vi "OpenVIFrontPanel.vi"(0 "VI Reference In":refnum<vi>, 5 "Wait Until Done (F)":bool, 7 "State(Standard)":T1(ring)=enum."Standard", 11 "error in":errorcluster) -> (4 "VI Reference Out":refnum<vi>, 15 "error out":errorcluster)   [LabVIEW 2016, in "Drona.lvlib" / "VI.lvlib"]
doc: "Opens the front panel of the VI by providing the VI reference."
uses:
  VI.lvlib
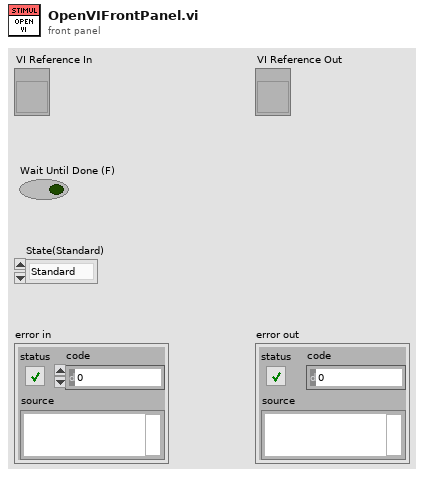
[diagram p1: front panel]
types:
  T1 = enum32{"Invalid", "Standard", "Closed", "Hidden", "Minimized", "Maximized"}
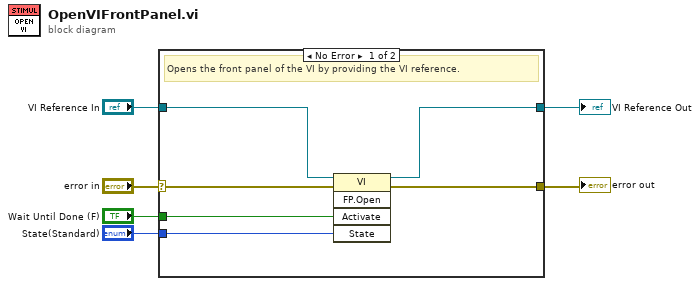
[diagram p0: block diagram]
diagram:
  n1 = case shown="No Error" "error in" {
    selector: "error in" -> [w8 w14]
    tunnel: "VI Reference In" -> [w11 w13]
    tunnel: [w10 w13] -> w4
    tunnel: [w12 w14] -> w3
    tunnel: "Wait Until Done (F)" -> [w9 _]
    tunnel: "State(Standard)" -> [w7 _]
    frame No Error {
      # "Opens the front panel of the VI by providing the VI reference."
      n2 = invoke on="Invoke Node" class="VI" method="FP.Open"(reference=w11, error in=w8, "Activate"=w9, "State"=w7) -> (reference out=w10:refnum<vi>, error out=w12:errorcluster)  [unwired: 1 in, 3 out]
    }
    frame Error {
    }
  }
  "error out" <- w3
  "VI Reference Out" <- w4
